vi "GE 5565PIORC.Registers.LAS1BA.Local Address Space 1 Base Address.Set.vi"(8 "error in (no error)":errorcluster, 10 "Local Address Space 1 Base Address":u32, 11 "GE 5565PIORC in":refnum<class "GE 5565PIORC.lvclass">) -> (0 "error out":errorcluster, 3 "GE 5565PIORC out":refnum<class "GE 5565PIORC.lvclass">)   [LabVIEW 2017, in "GE 5565PIORC.lvclass"]
doc: "The PCIBAR3 base address translates to the Local Address Space 1 Base Address programmed in this register. A Direct Slave access to an offset from PCIBAR3 maps to the same offset from this Local Base Address."
uses:
  GE 5565PIORC.lvclass
  GE 5565PIORC.Registers.Local Configuration.ctl
  GE 5565PIORC.lvclass/GE 5565PIORC.ctl
  GE 5565PIORC.Registers.Local Configuration.Read (U32).vi
  GE 5565PIORC.Registers.Local Configuration.Write (U32).vi
  Methods/GE 5565PIORC.Registers.Read.vi
  Methods/GE 5565PIORC.Registers.Read (U32).vi
  Methods/GE 5565PIORC.Registers.Write.vi
  Methods/GE 5565PIORC.Registers.Write (U32).vi
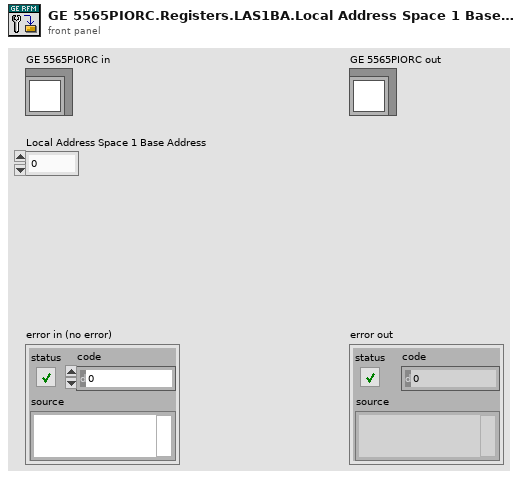
[diagram p1: front panel]
types:
  T1 = typedef "GE 5565PIORC.lvclass/GE 5565PIORC.Registers.Local Configuration.ctl" = u32
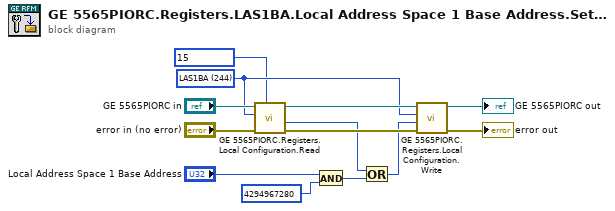
[diagram p0: block diagram]
diagram:
  w8 = T1 244 items=["MARBR"=8, "BIGEND"=12, "INTCSR"=104, "PCIHREV"=116, "DMAMODE0"=128, "DMAPADR0"=132, "DMALADR0"=136, "DMASIZ0"=140, "DMADPR0"=144, "DMACSR0"=168, "DMADAC0"=180, "LAS1RR"=240, "LAS1BA"=244] ("Local Configuration Registers")
  n1 = call-poly "GE 5565PIORC.Registers.Local Configuration.Read.vi"("Mask (0xFFFFFFFF)"=u32 15 ("y"), "error in (no error)"="error in (no error)", "Register"=w8, "GE 5565PIORC in"="GE 5565PIORC in") -> ("error out"=w5:errorcluster, "Value"=w3:u32, "GE 5565PIORC out"=w11:refnum<class "GE 5565PIORC.lvclass">)  [unwired: 5 in]
  n2 = And(x="Local Address Space 1 Base Address", y=u32 4294967280) -> (x .and. y?=w6:u32)
  n3 = Or(x=w3, y=w6) -> (x .or. y?=w4:u32)
  n4 = call-poly "GE 5565PIORC.Registers.Local Configuration.Write.vi"("error in (no error)"=w5, "Value"=w4, "Register"=w8, "GE 5565PIORC in"=w11) -> ("error out"=→"error out":errorcluster, "GE 5565PIORC out"=→"GE 5565PIORC out":refnum<class "GE 5565PIORC.lvclass">)  [unwired: 6 in]
